vi "Set Controls References Hash.vi"(8 "error in (no error)":errorcluster, 10 "Controls References Hash":variant, 11 "Hot And Cold Source Unit View in":refnum<class "Hot And Cold Source Unit View.lvclass">) -> (0 "error out":errorcluster, 3 "Hot And Cold Source Unit View out":refnum<class "Hot And Cold Source Unit View.lvclass">)   [LabVIEW 2013, in "Hot And Cold Source Unit View.lvlib" / "Hot And Cold Source Unit View.lvclass"]
uses:
  Hot And Cold Source Unit View.lvclass
  Hot And Cold Source Unit View.lvclass/Hot And Cold Source Unit View.ctl
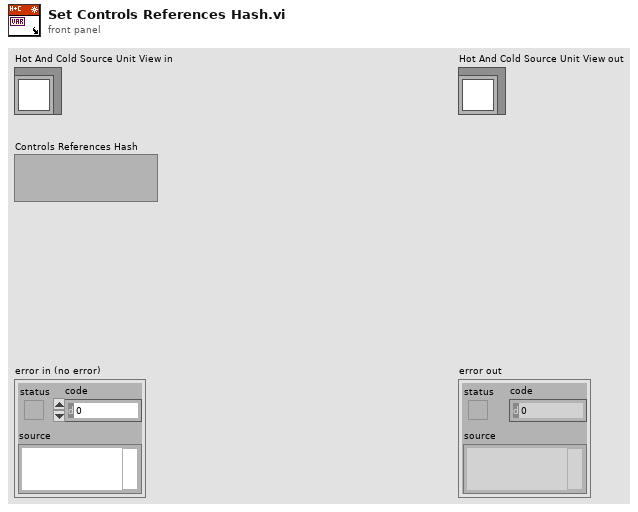
[diagram p1: front panel]
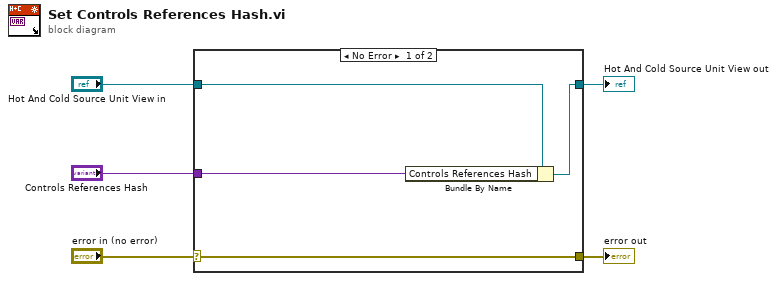
[diagram p0: block diagram]
diagram:
  n1 = case shown="No Error" "error in (no error)" {
    selector: "error in (no error)" -> [w9 w10]
    tunnel: [w9 w10] -> w4
    tunnel: [w7 w11] -> w2
    tunnel: "Hot And Cold Source Unit View in" -> [w8 w11]
    tunnel: "Controls References Hash" -> [w6 _]
    frame No Error {
      n2 = Bundle By Name(cluster=w8, "Controls References Hash"=w6) -> (w7:refnum<class "Hot And Cold Source Unit View.lvclass">)
    }
    frame Error {
    }
  }
  "error out" <- w4
  "Hot And Cold Source Unit View out" <- w2
